vi "20.1.-Data Socket Bidireccional 1.vi"() -> ()   [LabVIEW 2017]
panel:
  out "error out":errorcluster
  in  "stop":bool
  out "Boolean":bool
  in  "Slide":dbl(slide) scale=0.0..10.0
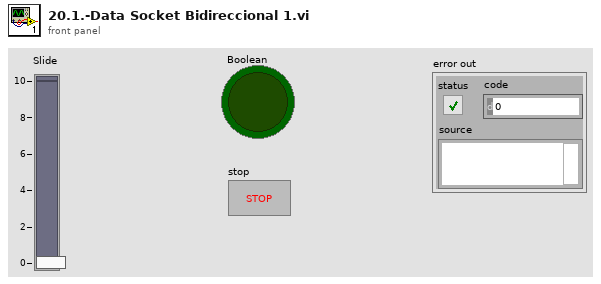
[diagram p1: front panel]
types:
  T1 = enum16{"Read", "Write", "ReadWrite", "BufferedRead", "BufferedReadWrite"}
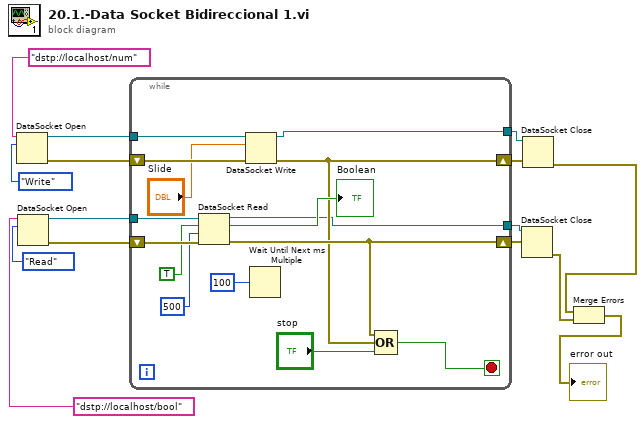
[diagram p0: block diagram]
diagram:
  n1 = DataSocket Open(10:T1."Write" ("mode"), 11:"dstp://localhost/num" ("URL")) -> (0:w14:errorcluster, 3:w15:refnum<k13>)  [unwired: 2 in]
  n2 = DataSocket Open(10:T1."Read" ("mode"), 11:"dstp://localhost/bool" ("URL")) -> (0:w12:errorcluster, 3:w13:refnum<k13>)  [unwired: 2 in]
  n3 = while {
    tunnel: w15 -> [w30]
    tunnel: w13 -> [w28]
    tunnel: [w18] -> w9
    tunnel: [w17] -> w8
    shift-right: [w21] -> w10
    shift-left: w14 -> [w29]
    shift-right: [w22] -> w11
    shift-left: w12 -> [w27]
    stop <- w19 stop-if-true
    n4 = DataSocket Read(8:w27, 9:500 ("ms timeout (10000)"), 10:TRUE, 11:w28) -> (0:w22:errorcluster, 2:→"Boolean":bool, 3:w17:refnum<k13>)  [unwired: 1 in, 4 out]
    n5 = DataSocket Write(8:w29, 10:"Slide", 11:w30) -> (0:w21:errorcluster, 3:w18:refnum<k13>)  [unwired: 1 in, 1 out]
    n6 = Wait Until Next ms Multiple(millisecond multiple=u32 100) -> ()  [unwired: 1 out]
    n7 = Compound Arithmetic op=OR(w22, w21, "stop") -> (w19:bool)
  }
  n8 = DataSocket Close(8:w11, 11:w8) -> (0:w2:errorcluster)  [unwired: 1 in, 1 out]
  n9 = DataSocket Close(8:w10, 11:w9) -> (0:w3:errorcluster)  [unwired: 1 in, 1 out]
  n10 = Merge Errors "Merge Errors"(w3, w2) -> (→"error out":errorcluster)
